vi "Terminal.vi"(8 "error in":errorcluster, 11 "refnum":refnum<vi>) -> (0 "error out":errorcluster, 3 "terminal":refnum<class "Terminal.lvclass">)   [LabVIEW 2014, in "Raspberry Pi Compatible Compiler for LabVIEW.lvlib" / "Terminal.lvclass"]
uses:
  Terminal.lvclass
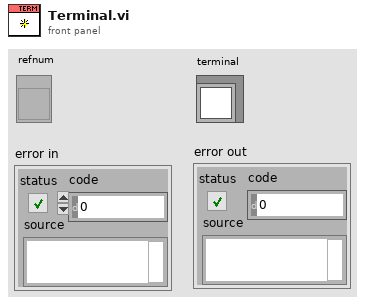
[diagram p1: front panel]
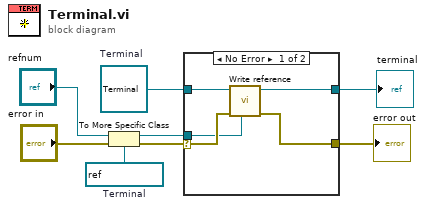
[diagram p0: block diagram]
diagram:
  w8 = refnum<vi> refnum  # Terminal
  w4 = refnum<class "Terminal.lvclass"> refnum  # Terminal
  n1 = To More Specific Class(target class=w8, reference="refnum", error in="error in") -> (specific class reference=w3:refnum<vi>, error out=w5:errorcluster)
  n2 = case shown="No Error" w5 {
    selector: w5 -> [w12 w15]
    tunnel: w4 -> [w13 w14]
    tunnel: w3 -> [w11 _]
    tunnel: [w10 w14] -> w1
    tunnel: [w9 w15] -> w2
    frame No Error {
      n3 = call-dynamic "Write reference.vi"("reference"=w11, "error in"=w12, "GObject in"=w13) -> ("error out"=w9:errorcluster, "GObject out"=w10:refnum<class "Terminal.lvclass">)  [unwired: 5 in]
    }
    frame Error {
    }
  }
  "error out" <- w2
  "terminal" <- w1
